vi "Add Class.vi"(8 "error in":errorcluster, 11 "Config in":refnum<class "Config.lvclass">) -> (0 "error out":errorcluster, 3 "Config out":refnum<class "Config.lvclass">)   [LabVIEW 2023, in "Config.lvlib" / "Config.lvclass"]
uses:
  Config.lvclass
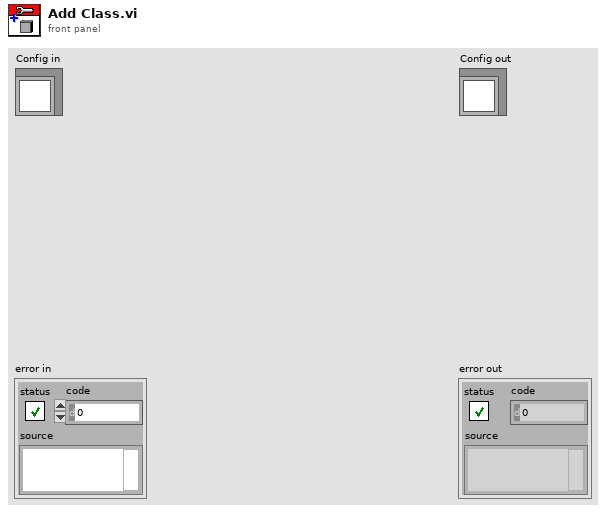
[diagram p1: front panel]
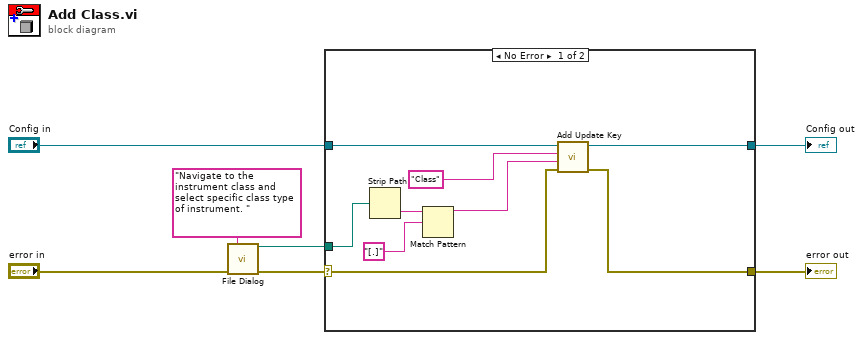
[diagram p0: block diagram]
diagram:
  n1 = call "File Dialog"("prompt"="Navigate to the instrument class and select specific class type of instrument. ", "error in"="error in") -> ("selected path"=w6:path, "error out"=w4:errorcluster)  [unwired: 10 in, 2 out]
  n2 = case shown="No Error" w4 {
    selector: w4 -> [w10 w17]
    tunnel: w6 -> [w14 _]
    tunnel: "Config in" -> [w13 w18]
    tunnel: [w12 w18] -> w3
    tunnel: [w9 w17] -> w2
    frame No Error {
      n3 = Strip Path(path=w14) -> (name=w15:string)  [unwired: 1 out]
      n4 = Match Pattern(string=w15, regular expression="[.]") -> (before substring=w8:string)  [unwired: 1 in, 3 out]
      n5 = call "Add Update Key.vi"("error in"=w10, "Value"=w8, "Key"="Class", "Config in"=w13) -> ("error out"=w9:errorcluster, "Config out"=w12:refnum<class "Config.lvclass">)  [unwired: 6 in]
    }
    frame Error {
    }
  }
  "error out" <- w2
  "Config out" <- w3
